vi "FTMS_alpha.vi"() -> ()   [LabVIEW 2011]
doc: "Enables and disables RF output of PSG1 & PSG2"
uses:
  LabVIEW/Hardware Control/OSC/SubVIs/controls/sampling_rate.ctl
  LabVIEW/Hardware Control/OSC/SubVIs/controls/scale.ctl
  LabVIEW/global.vi
panel:
  out "waiting":bool
  in  "Pause":bool
  in  "Stop":bool
  out "current step":i32
  out "current frequency":dbl format="%6.2p"
  out "current meas cycle":i32
  out "dt":dbl format="%#_6p"
  out "reset meas cycle timer":bool
  out "first start":bool
  in  "Tab Control":T1(tab)
  in  "EXP Meas Period (s)":dbl=10.0 min=1.0 format="%.2g"
  in  "Purge Freq.":dbl=2.0 caption="Purge Freq. (Hz)"
  in  "PURGE nozzle":bool
  in  "Refresh meas time":bool
  out "meas cycle time (ms)":u32
  in  "start experiment":bool
  in  "config TRIG":bool
  in  "config OSC":bool
  out "OSC resolution":ext=24999.999999999999998 caption="Resolution (Hz)" format="%#_6p"
  out "OSC sample points":i32=200000 caption="points / frame"
  out "TRIG BG cycle":dbl=100.0 caption="BG. cycle" min=0.0 max=999.999999999995 format="%.2p"
  out "TRIG mol delay":dbl=9.999999999999999e-05 caption="Mol. delay" min=0.0 max=999.999999999995 format="%.2p"
  out "TRIG start time":dbl[](array[numeric])=[0.0, 1.1e-06, 6.6e-06, 6.4e-06] caption="delay starts (s)" format="%.3p"
  out "TRIG burst enable":bool=TRUE caption="Burst"
  out "TRIG delay duration":dbl=4.6625e-05 caption="delay cycle (s)" format="%.2p"
  out "TRIG duration":dbl[](array[numeric])=[5.65e-06, 4.9999999999999996e-06, 4e-05, 4.9999999999999996e-06] caption="delay durations (s)" min=0.0 format="%.3p"
  out "TRIG burst period":dbl=4.9999999999999975e-05 caption="burst period (s)" format="%.2p"
  out "TRIG burst count":i32=1 caption="burst count"
  out "OSC hor scale":T2=4e-06 items=["400ns/div"=4e-07, "1µs/div"=1e-06, "2µs/div"=2e-06, "4µs/div"=4e-06, "10µs/div"=1e-05, "20µs/div"=2e-05]
  out "OSC sample rate":T3=5000000000.0 items=["20 GHz (50ps/sample)", "10 GHz (100ps/sample)", "5.0 GHz (200ps/sample)", "2.5 GHz (400ps/sample)", "1.25 GHz (0.8ns/sample)", "0.5 GHz (2ns/sample)"]
  in  "EXP Meas Cycles":i32=10 min=1 step=1
  in  "PSG start freq":dbl=0.0003 caption="Start Freq. (Hz)" min=0.00025 max=67.0 step=1e-06 format="%#.12p"
  in  "PSG Amplitude1":dbl caption="PSG1 Ampl (dBm)" min=-135.0 max=30.0 step=0.5 format="%#_8p"
  in  "PSG Amplitude 2":dbl caption="PSG2 Ampl (dBm)" min=-135.0 max=30.0 step=0.5 format="%#_8p"
  in  "PSG freq offset":dbl=0.0003 caption="freq. offset (Hz)" min=0.00025 max=67.0 step=1e-06 format="%#.12p"
  in  "write configs":bool
  in  "load config":bool
  in  "save config":bool
  in  "PSG steps":u32=1 min=1 step=1 format="%.0p"
  in  "PSG step size":dbl=0.0003 caption="step size" min=0.00025 max=67.0 step=1e-06 format="%#.12p"
  out "Meas Time":string="00:00:00"
  out "Experiment Time":string="00:00:00"
  in  "EXP chirp end":dbl=1000000000.0 format="%.2p"
  out "Current Molecular Frame":T4(graph) caption="Molecular Frame"
  out "Current Background Frame":T4(graph) caption="Background Frame"
  out "Current Cor Spectra":T4(graph) caption="Corrected Frame"
  out "frame averages completed:":i32 caption="averages:"
  in  "Frame":i32=1 caption="Displayed Frame" min=1 step=1
  in  "reset frame average":bool
  in  "frame single cycle":bool caption="no averaging"
  out "Average Cor":T4(graph) caption="Average of all corrected time domain signals"
  out "Averaged Background":T4(graph)
  out "Averaged Molecular":T4(graph)
  in  "Quit":bool
  # "local variables"
  # "General Settings"
  # "PSG Configuration"
  # "TRIG Configuration"
  # "OSC Configuration"
  # "File Storage"
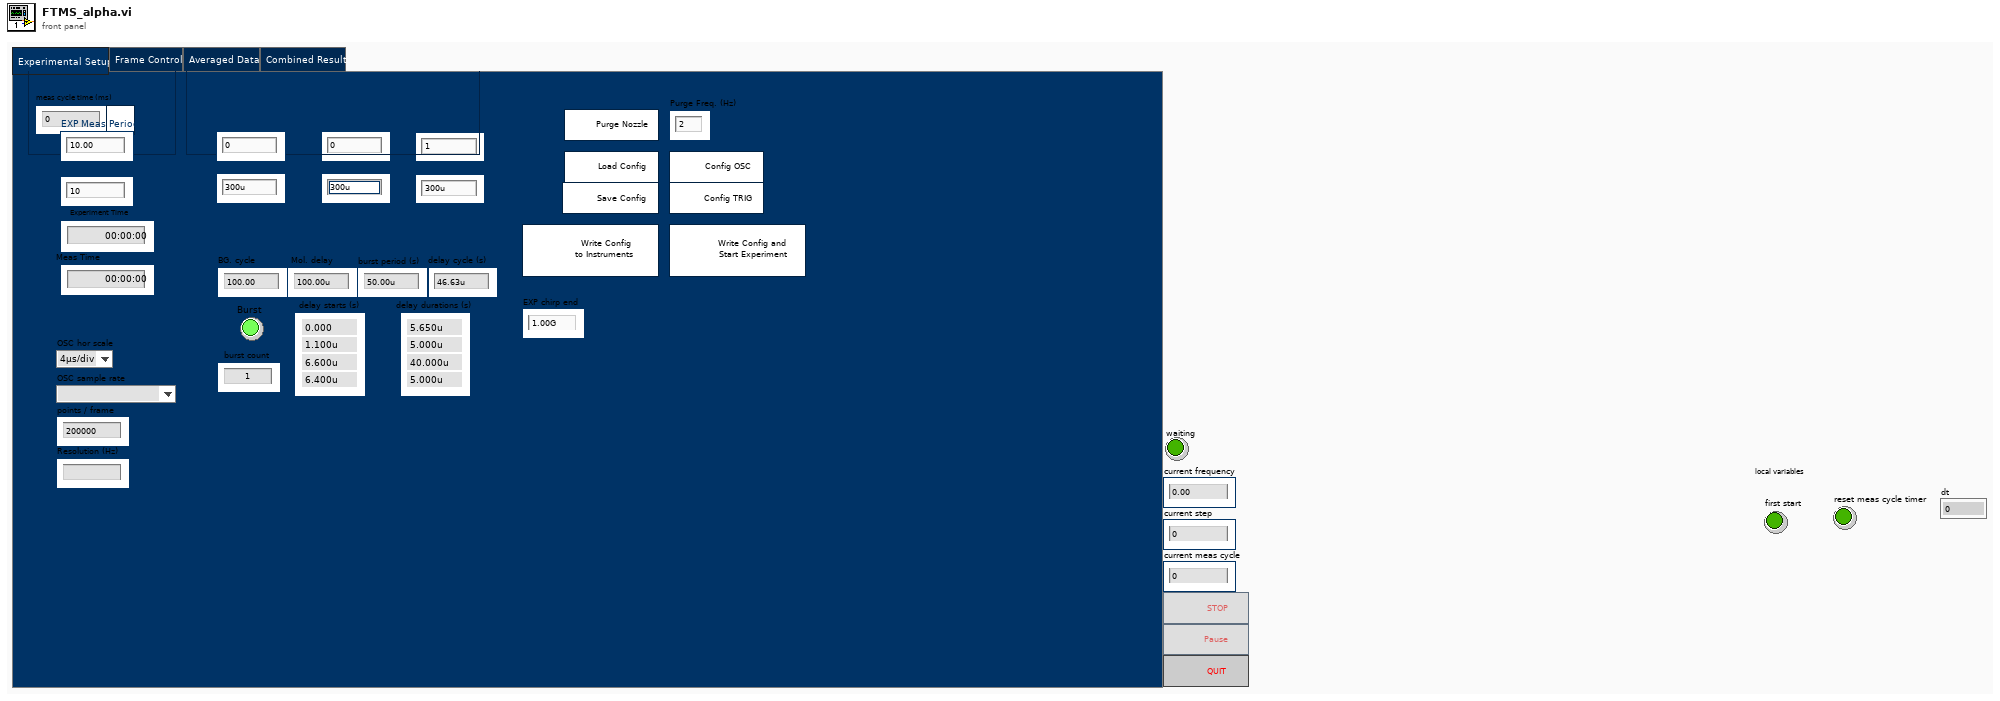
[diagram p1: front panel]
types:
  T1 = enum32{"Experimental Setup", "Frame Control", "Averaged Data", "Combined Result"}
  T2 = typedef "scale.ctl" = dbl
  T3 = typedef "sampling_rate.ctl" = ext
  T4 = cluster{"Numeric Control":dbl, "df":dbl, "magnitude":dbl[]}
  T5 = enum8{"Enabled", "Disabled", "Disabled and Grayed Out"}
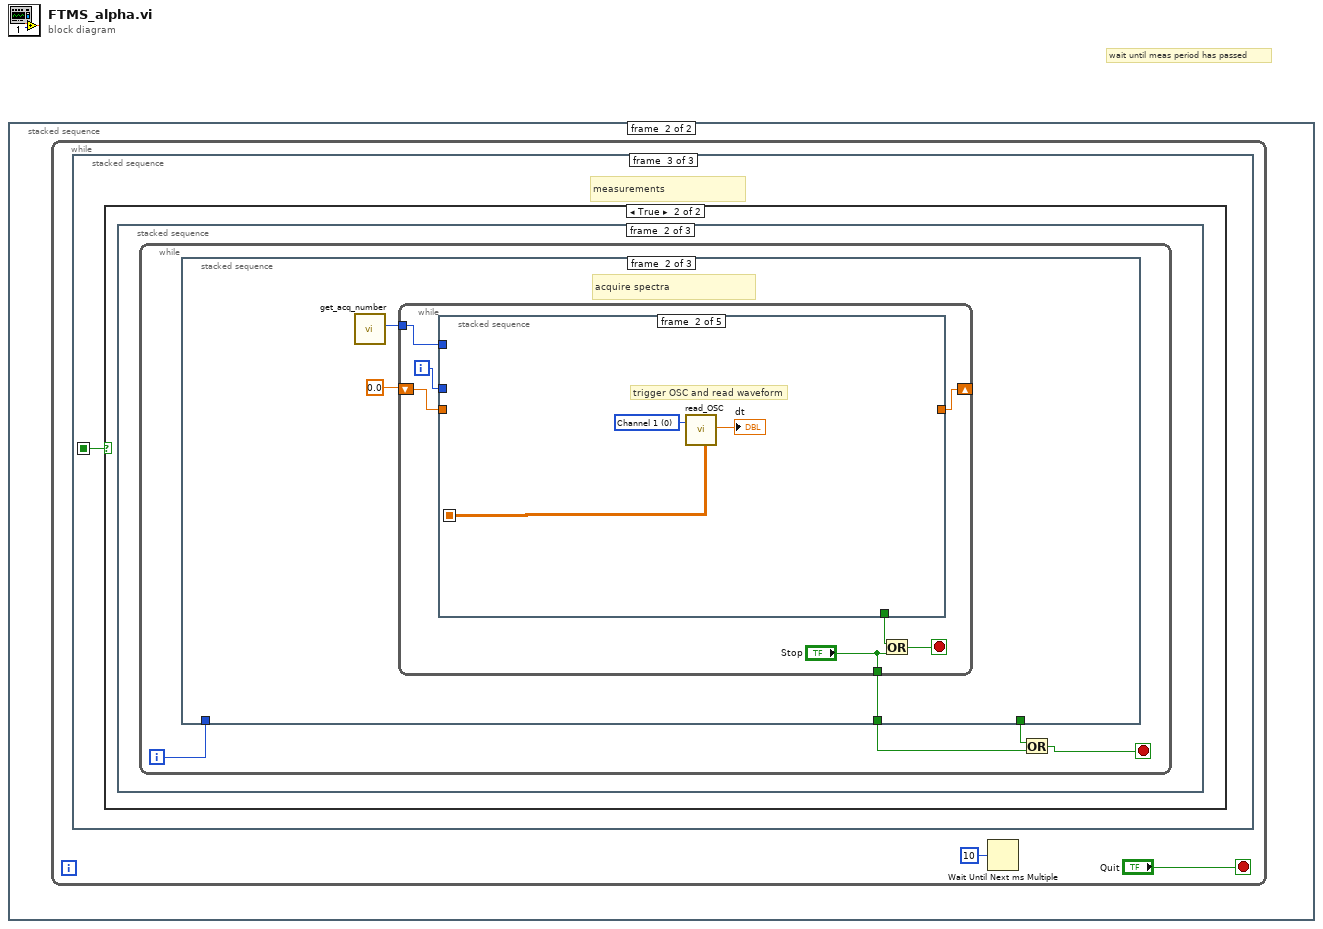
[diagram p0: block diagram]
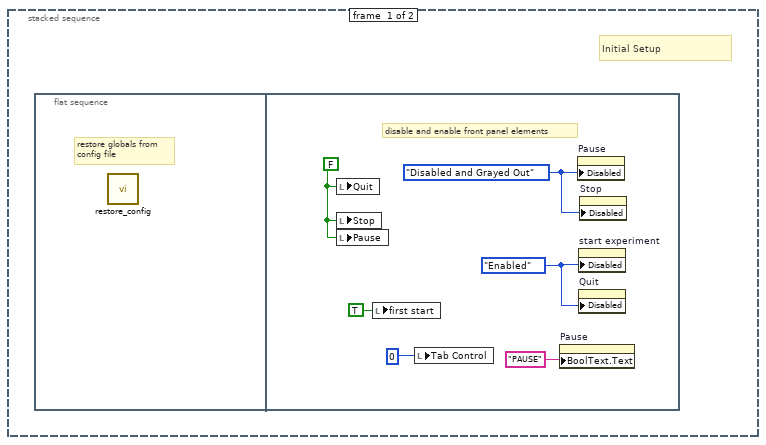
[diagram p2: hidden frame]
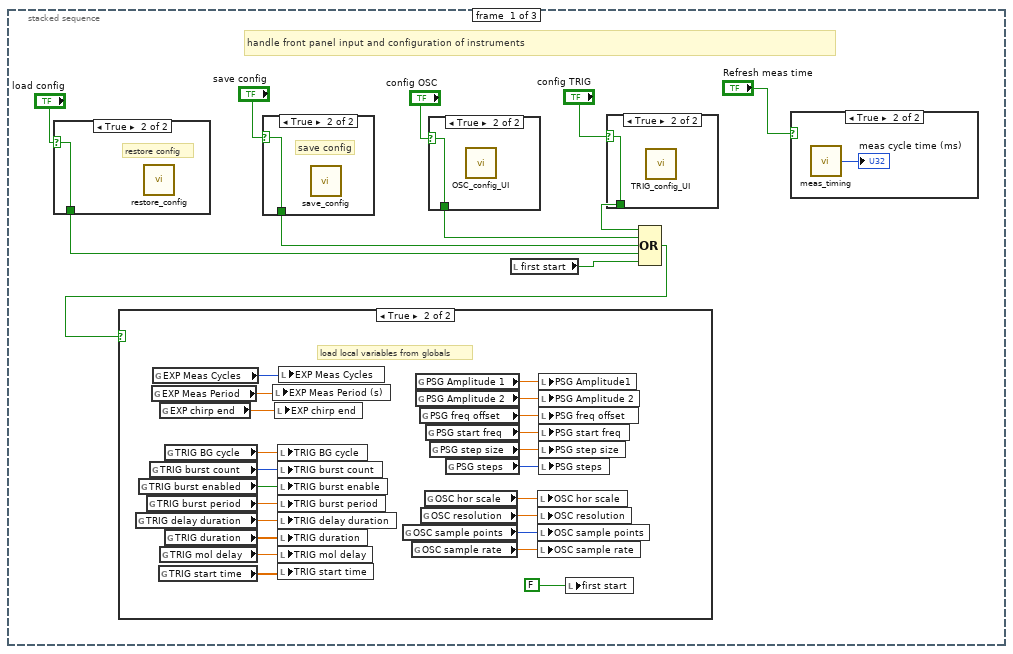
[diagram p3: hidden frame]
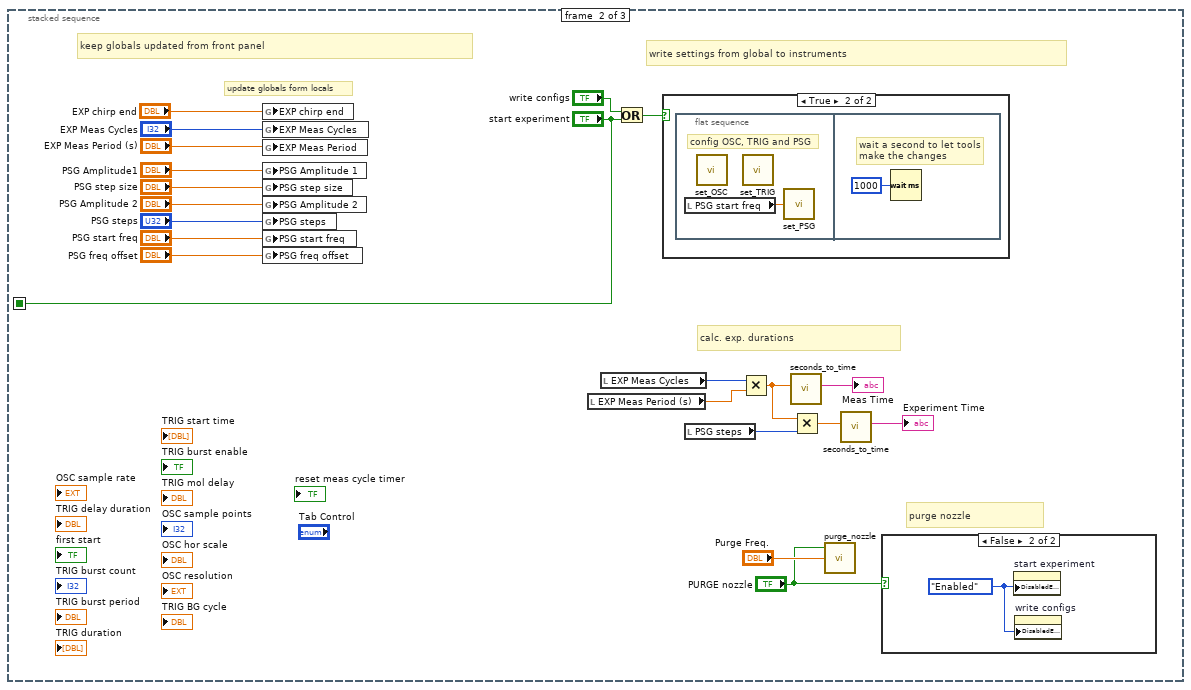
[diagram p10: hidden frame]
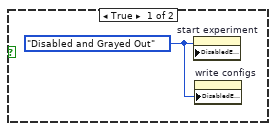
[diagram p11: hidden frame]
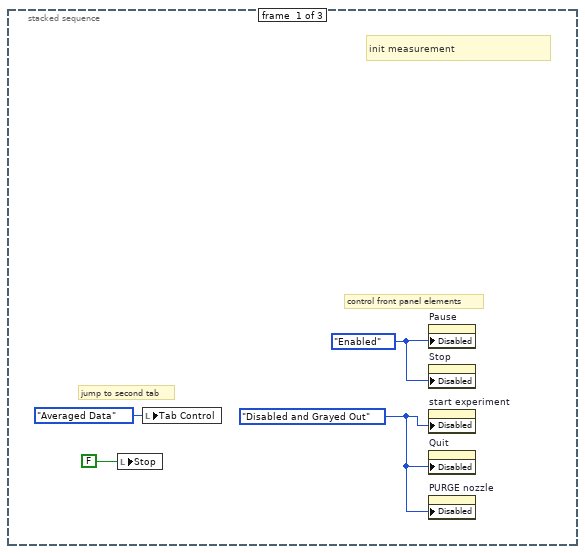
[diagram p14: hidden frame]
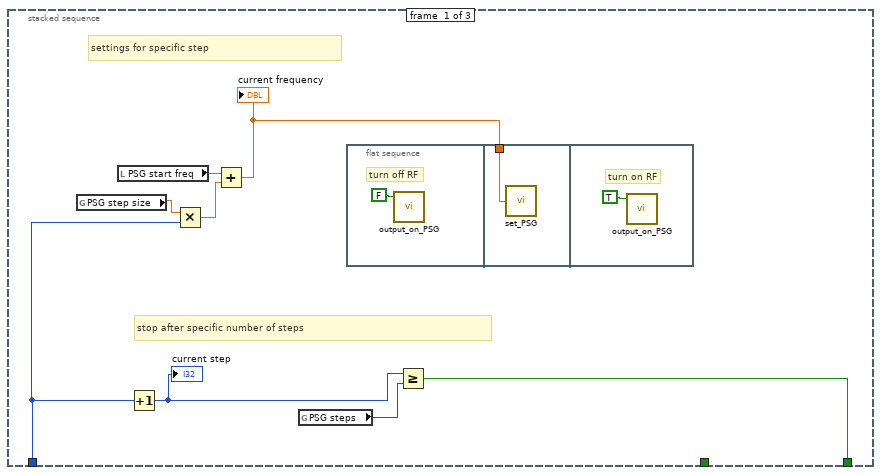
[diagram p15: hidden frame]
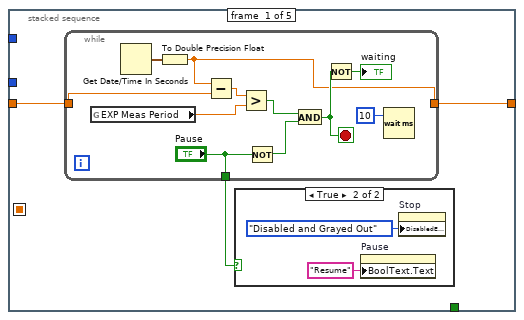
[diagram p16: hidden frame]
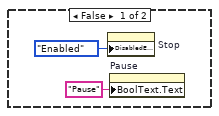
[diagram p17: hidden frame]
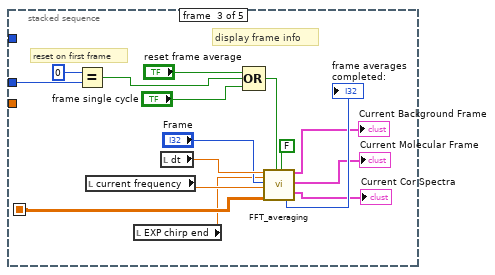
[diagram p18: hidden frame]
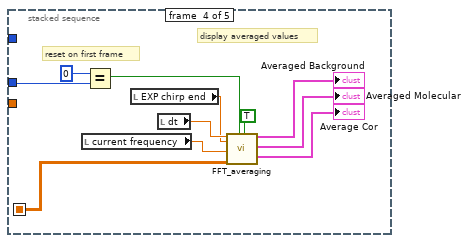
[diagram p19: hidden frame]
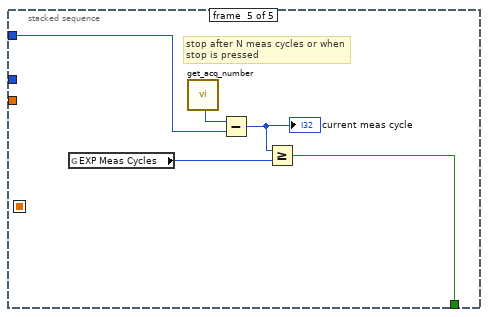
[diagram p20: hidden frame]
diagram:
  # "wait until meas period has passed"
  n1 = stacked-sequence {
    frame #0 {
      # "Initial Setup"
      n2 = flat-sequence {
        frame #0 {
          # "restore globals from\nconfig file"
          n3 = call "restore_config.vi"() -> ()  [unwired: 5 in]
        }
        frame #1 {
          w5 = T5."Disabled and Grayed Out" ("Disabled")
          w2 = T5."Enabled" ("Disabled")
          w6 = FALSE ("Quit")
          # "disable and enable front panel elements"
          n4 = local write "Quit"(w6) -> ()
          n5 = local write "Stop"(w6) -> ()
          n6 = local write "Pause"(w6) -> ()
          n7 = local write "first start"(TRUE ("first start")) -> ()
          n8 = local write "Tab Control"(0) -> ()
          n9 = property on="Pause" class="Bool (strict)"("BoolText.Text"="PAUSE" ("Boolean Text.Text")) -> ()  [unwired: 2 in, 2 out]
          n10 = property on="Pause" class="Bool (strict)"("Disabled"=w5) -> ()  [unwired: 2 in, 2 out]
          n11 = property on="start experiment" class="Bool"("Disabled"=w2) -> ()  [unwired: 2 in, 2 out]
          n12 = property on="Quit" class="Bool (strict)"("Disabled"=w2) -> ()  [unwired: 2 in, 2 out]
          n13 = property on="Stop" class="Bool (strict)"("Disabled"=w5) -> ()  [unwired: 2 in, 2 out]
        }
      }
    }
    frame #1 {
      n14 = while {
        stop <- "Quit" stop-if-true
        n15 = stacked-sequence {
          seq-local: [_ "start experiment" _] -> [_ _ w76]
          frame #0 {
            # "handle front panel input and configuration of instruments"
            n16 = case shown="True" "load config" {
              selector: "load config" -> [w49 w50]
              tunnel: [w49 w50] -> w11
              frame False {
              }
              frame True {
                # "restore config"
                n17 = call "restore_config.vi"() -> ()  [unwired: 5 in]
              }
            }
            n18 = case shown="True" "save config" {
              selector: "save config" -> [w47 w48]
              tunnel: [w47 w48] -> w13
              frame False {
              }
              frame True {
                # "save config"
                n19 = call "save_config.vi"() -> ()  [unwired: 5 in]
              }
            }
            n20 = case shown="True" "config OSC" {
              selector: "config OSC" -> [w45 w46]
              tunnel: [w45 w46] -> w15
              frame False {
              }
              frame True {
                n21 = call "OSC_config_UI.vi"() -> ()  [unwired: 12 in]
              }
            }
            n22 = local read "first start"() -> (w18:bool)
            n23 = case shown="True" "config TRIG" {
              selector: "config TRIG" -> [w43 w44]
              tunnel: [w43 w44] -> w16
              frame False {
              }
              frame True {
                n24 = call "TRIG_config_UI.vi"() -> ()  [unwired: 12 in]
              }
            }
            n25 = Compound Arithmetic op=OR(w16, w15, w13, w11, w18) -> (w10:bool)
            n26 = case shown="True" w10 {
              frame False {
              }
              frame True {
                # "load local variables from globals"
                n27 = global read "global.vi" "TRIG delay duration"() -> (w28:dbl)
                n28 = global read "global.vi" "TRIG burst enabled"() -> (w30:bool)
                n29 = global read "global.vi" "TRIG burst period"() -> (w29:dbl)
                n30 = global read "global.vi" "TRIG burst count"() -> (w31:i32)
                n31 = global read "global.vi" "EXP Meas Period"() -> (w23:dbl)
                n32 = global read "global.vi" "EXP Meas Cycles"() -> (w42:i32)
                n33 = global read "global.vi" "TRIG start time"() -> (w25:dbl[])
                n34 = global read "global.vi" "EXP chirp end"() -> (w21:dbl)
                n35 = global read "global.vi" "TRIG mol delay"() -> (w26:dbl)
                n36 = global read "global.vi" "TRIG BG cycle"() -> (w32:dbl)
                n37 = global read "global.vi" "TRIG duration"() -> (w27:dbl[])
                n38 = local write "EXP Meas Period (s)"(w23) -> ()
                n39 = local write "EXP chirp end"(w21) -> ()
                n40 = local write "TRIG BG cycle"(w32) -> ()
                n41 = local write "TRIG burst count"(w31) -> ()
                n42 = local write "TRIG burst enable"(w30) -> ()
                n43 = local write "TRIG burst period"(w29) -> ()
                n44 = local write "TRIG delay duration"(w28) -> ()
                n45 = local write "TRIG duration"(w27) -> ()
                n46 = local write "TRIG mol delay"(w26) -> ()
                n47 = local write "TRIG start time"(w25) -> ()
                n48 = local write "EXP Meas Cycles"(w42) -> ()
                n49 = global read "global.vi" "OSC sample points"() -> (w40:i32)
                n50 = global read "global.vi" "OSC sample rate"() -> (w39:T3)
                n51 = global read "global.vi" "PSG Amplitude 1"() -> (w34:dbl)
                n52 = global read "global.vi" "PSG Amplitude 2"() -> (w35:dbl)
                n53 = global read "global.vi" "PSG freq offset"() -> (w36:dbl)
                n54 = global read "global.vi" "OSC resolution"() -> (w41:ext)
                n55 = global read "global.vi" "OSC hor scale"() -> (w22:T2)
                n56 = global read "global.vi" "PSG start freq"() -> (w37:dbl)
                n57 = global read "global.vi" "PSG step size"() -> (w38:dbl)
                n58 = global read "global.vi" "PSG steps"() -> (w33:i32)
                n59 = local write "OSC hor scale"(w22) -> ()
                n60 = local write "OSC resolution"(w41) -> ()
                n61 = local write "OSC sample points"(w40) -> ()
                n62 = local write "OSC sample rate"(w39) -> ()
                n63 = local write "PSG Amplitude1"(w34) -> ()
                n64 = local write "PSG Amplitude 2"(w35) -> ()
                n65 = local write "PSG freq offset"(w36) -> ()
                n66 = local write "PSG start freq"(w37) -> ()
                n67 = local write "PSG step size"(w38) -> ()
                n68 = local write "PSG steps"(w33) -> ()
                n69 = local write "first start"(FALSE ("first start")) -> ()
              }
            }
            n70 = case shown="True" "Refresh meas time" {
              frame False {
              }
              frame True {
                n71 = call "meas_timing.vi"() -> ("meas cycle time"=→"meas cycle time (ms)":u32)  [unwired: 5 in]
              }
            }
          }
          frame #1 {
            # "calc. exp. durations"
            # "purge nozzle"
            # "write settings from global to instruments"
            # "keep globals updated from front panel"
            # "update globals form locals"
            n72 = global write "global.vi" "EXP chirp end"("EXP chirp end") -> ()
            n73 = global write "global.vi" "EXP Meas Cycles"("EXP Meas Cycles") -> ()
            n74 = global write "global.vi" "EXP Meas Period"("EXP Meas Period (s)") -> ()
            n75 = global write "global.vi" "PSG Amplitude 1"("PSG Amplitude1") -> ()
            n76 = global write "global.vi" "PSG step size"("PSG step size") -> ()
            n77 = global write "global.vi" "PSG Amplitude 2"("PSG Amplitude 2") -> ()
            n78 = global write "global.vi" "PSG steps"("PSG steps") -> ()
            n79 = global write "global.vi" "PSG start freq"("PSG start freq") -> ()
            n80 = global write "global.vi" "PSG freq offset"("PSG freq offset") -> ()
            n81 = local read "EXP Meas Period (s)"() -> (w58:dbl)
            n82 = local read "EXP Meas Cycles"() -> (w59:i32)
            n83 = Or(x="write configs", y="start experiment") -> (x .or. y?=w63:bool)
            n84 = case shown="True" w63 {
              frame False {
              }
              frame True {
                n85 = flat-sequence {
                  frame #0 {
                    # "config OSC, TRIG and PSG"
                    n86 = local read "PSG start freq"() -> (w74:dbl)
                    n87 = call "set_OSC.vi"() -> ()  [unwired: 12 in]
                    n88 = call "set_TRIG.vi"() -> ()  [unwired: 12 in]
                    n89 = call "set_PSG.vi"("PSG1 frequency"=w74) -> ()  [unwired: 5 in]
                  }
                  frame #1 {
                    # "wait a second to let tools \nmake the changes"
                    n90 = Wait (ms)(milliseconds to wait=u32 1000) -> ()  [unwired: 1 out]
                  }
                }
              }
            }
            n91 = local read "PSG steps"() -> (w55:u32)
            n92 = Multiply(x=w59, y=w58) -> (x*y=w56:dbl)
            n93 = call "seconds_to_time.vi"("# Seconds (0)"=w56) -> ("Elapsed Time (00:00:00)"=→"Meas Time":string)  [unwired: 10 in]
            n94 = Multiply(x=w56, y=w55) -> (x*y=w53:dbl)
            n95 = call "purge_nozzle.vi"("purge frequency"="Purge Freq.", "Purge"="PURGE nozzle") -> ()  [unwired: 4 in]
            n96 = call "seconds_to_time.vi"("# Seconds (0)"=w53) -> ("Elapsed Time (00:00:00)"=→"Experiment Time":string)  [unwired: 10 in]
            n97 = case shown="False" "PURGE nozzle" {
              frame True {
                w72 = T5."Disabled and Grayed Out" ("Disabled")
                n98 = property on="start experiment" class="Bool"("DisabledEnum"=w72) -> ()  [unwired: 2 in, 2 out]
                n99 = property on="write configs" class="Bool"("DisabledEnum"=w72) -> ()  [unwired: 2 in, 2 out]
              }
              frame False {
                w73 = T5."Enabled" ("Disabled")
                n100 = property on="start experiment" class="Bool"("DisabledEnum"=w73) -> ()  [unwired: 2 in, 2 out]
                n101 = property on="write configs" class="Bool"("DisabledEnum"=w73) -> ()  [unwired: 2 in, 2 out]
              }
            }
          }
          frame #2 {
            # "measurements"
            n102 = case shown="True" w76 {
              frame False {
              }
              frame True {
                n103 = stacked-sequence {
                  frame #0 {
                    w80 = T5."Enabled" ("Disabled")
                    w79 = T5."Disabled and Grayed Out" ("Disabled")
                    # "init measurement"
                    # "control front panel elements"
                    # "jump to second tab"
                    n104 = local write "Stop"(FALSE ("Stop")) -> ()
                    n105 = local write "Tab Control"(T1."Averaged Data" ("Tab Control")) -> ()
                    n106 = property on="Pause" class="Bool (strict)"("Disabled"=w80) -> ()  [unwired: 2 in, 2 out]
                    n107 = property on="Stop" class="Bool (strict)"("Disabled"=w80) -> ()  [unwired: 2 in, 2 out]
                    n108 = property on="start experiment" class="Bool"("Disabled"=w79) -> ()  [unwired: 2 in, 2 out]
                    n109 = property on="Quit" class="Bool (strict)"("Disabled"=w79) -> ()  [unwired: 2 in, 2 out]
                    n110 = property on="PURGE nozzle" class="Bool (strict)"("Disabled"=w79) -> ()  [unwired: 2 in, 2 out]
                  }
                  frame #1 {
                    n111 = while {
                      i -> [w84]
                      stop <- w82 stop-if-true
                      n112 = stacked-sequence {
                        tunnel: w84 -> [w89 _ _]
                        tunnel: [w88 _ _] -> w83
                        tunnel: [_ w96 _] -> w81
                        frame #0 {
                          # "stop after specific number of steps"
                          # "settings for specific step"
                          n113 = global read "global.vi" "PSG step size"() -> (w92:dbl)
                          n114 = local read "PSG start freq"() -> (w91:dbl)
                          n115 = Increment(x=w89) -> (x+1=w86:i32)
                          "current step" <- w86
                          n116 = Multiply(x=w92, y=w89) -> (x*y=w90:dbl)
                          n117 = Add(x=w91, y=w90) -> (x+y=w85:dbl)
                          "current frequency" <- w85
                          n118 = global read "global.vi" "PSG steps"() -> (w87:i32)
                          n119 = flat-sequence {
                            tunnel: w85 -> [w94]
                            frame #0 {
                              # "turn off RF"
                              n120 = call "output_on_PSG.vi"("Enable RF Output (F:Disable)"=FALSE) -> ()  [unwired: 5 in]
                            }
                            frame #1 {
                              n121 = call "set_PSG.vi"("PSG1 frequency"=w94) -> ()  [unwired: 5 in]
                            }
                            frame #2 {
                              # "turn on RF"
                              n122 = call "output_on_PSG.vi"("Enable RF Output (F:Disable)"=TRUE) -> ()  [unwired: 5 in]
                            }
                          }
                          n123 = Greater Or Equal?(x=w86, y=w87) -> (x >= y?=w88:bool)
                        }
                        frame #1 {
                          # "acquire spectra"
                          n124 = call "get_acq_number.vi"() -> ("# of meas cycles"=w97:i32)  [unwired: 8 in, 3 out]
                          n125 = while {
                            tunnel: w97 -> [w104]
                            shift-right: [w102] -> _
                            shift-left: 0.0 -> [w101]
                            tunnel: ["Stop"] -> w96
                            i -> [w105]
                            stop <- w100 stop-if-true
                            n126 = stacked-sequence {
                              seq-local: [_ w126 _ _ _] -> [_ _ w135 w147 _]
                              tunnel: w105 -> [_ _ w137 w151 _]
                              tunnel: w104 -> [_ _ _ _ w157]
                              tunnel: [_ _ _ _ w156] -> w103
                              tunnel: [w108 _ _ _ _] -> w102
                              tunnel: w101 -> [w107 _ _ _ _]
                              frame #0 {
                                n127 = while {
                                tunnel: [w116] -> w108
                                tunnel: w107 -> [w122]
                                tunnel: ["Pause"] -> w106
                                stop <- w118 stop-if-true
                                n128 = global read "global.vi" "EXP Meas Period"() -> (w120:dbl)
                                n129 = Get Date/Time In Seconds() -> (seconds since 1Jan1904=w123:timestamp)
                                n130 = To Double Precision Float(number=w123) -> (double precision float=w116:dbl)
                                n131 = Subtract(x=w116, y=w122) -> (x-y=w121:dbl)
                                n132 = Greater?(x=w121, y=w120) -> (0:w115:bool)
                                n133 = Not(x="Pause") -> (.not. x?=w114:bool)
                                n134 = And(x=w115, y=w114) -> (x .and. y?=w118:bool)
                                n135 = Not(x=w118) -> (.not. x?=→"waiting":bool)
                                n136 = Wait (ms)(milliseconds to wait=u32 10) -> ()  [unwired: 1 out]
                                }
                                n137 = case shown="True" w106 {
                                frame False {
                                n138 = property on="Stop" class="Bool (strict)"("DisabledEnum"=T5."Enabled" ("Disabled")) -> ()  [unwired: 2 in, 2 out]
                                n139 = property on="Pause" class="Bool (strict)"("BoolText.Text"="Pause" ("Caption.Text")) -> ()  [unwired: 2 in, 2 out]
                                }
                                frame True {
                                n140 = property on="Pause" class="Bool (strict)"("BoolText.Text"="Resume" ("Caption.Text")) -> ()  [unwired: 2 in, 2 out]
                                n141 = property on="Stop" class="Bool (strict)"("DisabledEnum"=T5."Disabled and Grayed Out" ("Disabled")) -> ()  [unwired: 2 in, 2 out]
                                }
                                }
                              }
                              frame #1 {
                                w125 = u16 0 items=["Channel 1", "Channel 2", "Channel 3", "Channel 4", "Math 1", "Math 2", "Math 3", "Math 4", "Reference 1", "Reference 2", "Reference 3", "Reference 4"] ("Channel (0: Channel 1)")
                                # "trigger OSC and read waveform"
                                n142 = call "read_OSC.vi"("Channel (0: Channel 1)"=w125) -> ("appended array"=w126:dbl[][][], "dt"=→"dt":dbl)  [unwired: 7 in, 2 out]
                              }
                              frame #2 {
                                # "reset on first frame"
                                # "display frame info"
                                n143 = Equal?(x=0, y=w137) -> (x = y?=w133:bool)
                                n144 = local read "current frequency"() -> (w141:dbl)
                                n145 = local read "EXP chirp end"() -> (w127:dbl)
                                n146 = local read "dt"() -> (w142:dbl)
                                n147 = Compound Arithmetic op=OR("reset frame average", w133, "frame single cycle") -> (w131:bool)
                                n148 = call "FFT_averaging.vi"("dt"=w142, "chirp end"=w127, "frame"="Frame", "current frequency"=w141, "3d waveform array"=w135, "reset frame average"=w131, "all frames?"=FALSE) -> ("averages compl"=→"frame averages completed:":i32, "BG spectrum"=→"Current Background Frame":T4, "Mol spectrum"=→"Current Molecular Frame":T4, "cor spectrum"=→"Current Cor Spectra":T4)  [unwired: 6 in, 3 out]
                              }
                              frame #3 {
                                # "reset on first frame"
                                # "display averaged values"
                                n149 = local read "current frequency"() -> (w149:dbl)
                                n150 = Equal?(x=0, y=w151) -> (x = y?=w148:bool)
                                n151 = local read "EXP chirp end"() -> (w144:dbl)
                                n152 = local read "dt"() -> (w150:dbl)
                                n153 = call "FFT_averaging.vi"("dt"=w150, "chirp end"=w144, "current frequency"=w149, "3d waveform array"=w147, "reset frame average"=w148, "all frames?"=TRUE) -> ("BG spectrum"=→"Averaged Background":T4, "Mol spectrum"=→"Averaged Molecular":T4, "cor spectrum"=→"Average Cor":T4)  [unwired: 7 in, 4 out]
                              }
                              frame #4 {
                                # "stop after N meas cycles or when \nstop is pressed"
                                n154 = global read "global.vi" "EXP Meas Cycles"() -> (w154:i32)
                                n155 = call "get_acq_number.vi"() -> ("# of meas cycles"=w158:i32)  [unwired: 8 in, 3 out]
                                n156 = Subtract(x=w158, y=w157) -> (x-y=w155:i32)
                                "current meas cycle" <- w155
                                n157 = Greater Or Equal?(x=w155, y=w154) -> (x >= y?=w156:bool)
                              }
                            }
                            n158 = Or(x=w103, y="Stop") -> (x .or. y?=w100:bool)
                          }
                        }
                        frame #2 {
                          # "save between steps as backup, overwrite old files"
                        }
                      }
                      n159 = Or(x=w83, y=w81) -> (x .or. y?=w82:bool)
                    }
                  }
                  frame #2 {
                    w162 = T5."Disabled and Grayed Out" ("Disabled")
                    w161 = T5."Enabled" ("Disabled")
                    # "turn off RF"
                    n160 = local write "Stop"(FALSE ("Stop")) -> ()
                    n161 = call "output_on_PSG.vi"("Enable RF Output (F:Disable)"=FALSE) -> ()  [unwired: 5 in]
                    n162 = property on="Pause" class="Bool (strict)"("Disabled"=w162) -> ()  [unwired: 2 in, 2 out]
                    n163 = property on="Stop" class="Bool (strict)"("Disabled"=w162) -> ()  [unwired: 2 in, 2 out]
                    n164 = property on="start experiment" class="Bool"("Disabled"=w161) -> ()  [unwired: 2 in, 2 out]
                    n165 = property on="Quit" class="Bool (strict)"("Disabled"=w161) -> ()  [unwired: 2 in, 2 out]
                    n166 = property on="PURGE nozzle" class="Bool (strict)"("Disabled"=w161) -> ()  [unwired: 2 in, 2 out]
                  }
                }
              }
            }
          }
        }
        n167 = Wait Until Next ms Multiple(millisecond multiple=u32 10) -> ()  [unwired: 1 out]
      }
    }
  }
